vi "beads_DAQ_tmp.vi"() -> ()   [LabVIEW 2018]
panel:
  in  "Set Leak":bool
  out "apparent_leak_rate":dbl=8.332270636437045e-10
  in  "desired_leak_rate (torr*l/s)":dbl format="%.2e"
  out "P_baratron [torr]":dbl=6.441508062591926e-05 format="%#_3g"
  out "P_pirani [torr]":dbl=9.08455806667689e-05 format="%#_3g"
  out "P_1Tbaratro [torr]":dbl=8.203640319307528e-05 format="%#_3g"
  out "T_elec_rack [C]":dbl
  out "T_opt_table [C]":dbl
  in  "Read pressures?":bool=TRUE
  in  "Read temps?":bool
  in  "img_cluster":cluster{"Take Pic?":bool, "Only Images":bool}
  in  "Picomotor Stepping":T1={"Motor 1 Step Size"=-2, "zig zag iterations"=0, "Motor 2 Step Size"=0, "Step Picomotors?"=FALSE, "td (ms)"=0.0, "num"=0}
  in  "signal type":T2(ring)
  in  "Add small amp?":bool
  in  "Small amp freq (Hz)":dbl=10.0 format="%0.2p"
  in  "Small amp":dbl=1.0 format="%0.2p"
  in  "Flash lamp\n settings:":T3={"Flash lamp?"=FALSE, "Number of cyles\nbetween flashes"=2, "# Pulses"=2, "Stop flashing \nbelow thresh?"=TRUE, "Stop threshold"=25.0, "Pulse voltage?"=FALSE, "Pulse length (ms)"=0.001, "Pulse amp (V)"=0.001, "Disable AWG"=FALSE}
  in  "Stage settings:":T4={"Set stage?"=FALSE, "start X (um)"=40.0, "stop X (um) "=40.0, "# X Steps"=1, "start Y (um)"=40.0, "stop Y (um) "=40.0, "# Y steps"=1, "start Z (um)"=80.0, "stop Z (um)"=80.0, "# Z steps "=1, "Swp X?"=FALSE, "Amplitude X (um)"=40.0, "Frequency X (Hz)"=10.0, "Amplitude Y (um)"=40.0, "Frequency Y (Hz)"=3.7, "Amplitude Z (um)"=10.0, "Frequency Z (Hz)"=17.0, "Swp Y?"=FALSE, "Swp Z?"=FALSE}
  in  "Electrode settings:":T5={"DC volts (V):\n"=[0.0, 0.0, 0.0, 0.0, 0.0, 0.0, 0.0, 0.0], "Electrode to sweep:"=3, "start volt (V)"=4.0, "stop volt (V) "=4.0, "# V Steps"=1, "start freq (Hz)"=41.0, "stop freq (Hz) "=41.0, "# F steps"=1, "start DC (V)"=0.0, "stop DC (V)"=0.0, "# DC steps "=1, "Digitize electrode\ndrives?"=TRUE, "Sweep electrode?"=FALSE, "Add 0.5*V DC \noffset for amp?"=FALSE, "Use electrode \nconfig file?"=FALSE, "Path"=path "C:/GitHub/opt_lev/labview/DAQ_settings/electrode_sweep.txt", "Use arbitrary\nforce func?"=FALSE, "Voltage vs pos file"=path "C:/GitHub/opt_lev/labview/DAQ_settings/electrode_sweep.txt", "Use Arbitray\nelec drive"=FALSE, "Elec Drive File"=path "C:/GitHub/opt_lev_controls/labview/DAQ_settings/freq_comb_elec3_10V_1-600Hz_nocutsamp.txt", "Filter Elecs?"=FALSE, "Filter Cantilever?"=FALSE, "Control DDS"=TRUE, "x bias start (V)"=0.02, "x bias stop (V)"=-0.02, "y bias start (V)"=0.0, "y bias stop (V)"=0.0, "z bias start (V)"=0.0, "z bias stop (V)"=0.0}
  in  "DC supply settings:":T6
  out "Data":dbl[][](graph)
  out "Curr threshold":dbl=0.44040576014655786
  in  "Number of Samples":i32=50000
  in  "Sample Rate [Hz]":dbl=5000.0
  out "Actual Sample \nRate":dbl=5000.0 format="%0.2f"
  in  "Delay between files [s]":dbl=4.0 caption="Delay Time (s)"
  in  "Num files":i32=500
  in  "File base name":string="turbombar_powfb_xyzcool"
  in  "Directory path":path=path "D:/data/20210521/bead1/neutrality/w_height_fb_100V_41_Hz_bias_sweep_y_slow_dds_100kHz_spinning_xz"
  # "Logging Settings"
  # "Environment"
  # "Picomotor Stepping"
  # "Flash Lamp Settings"
  # "1: -35, 2: -30\n\n1: 32  2: 30"
  # "0"
  # "1"
  # "2"
  # "3"
  # "4"
  # "5"
  # "6"
  # "7"
  # "Acquired Data"
  # "Timing Settings"
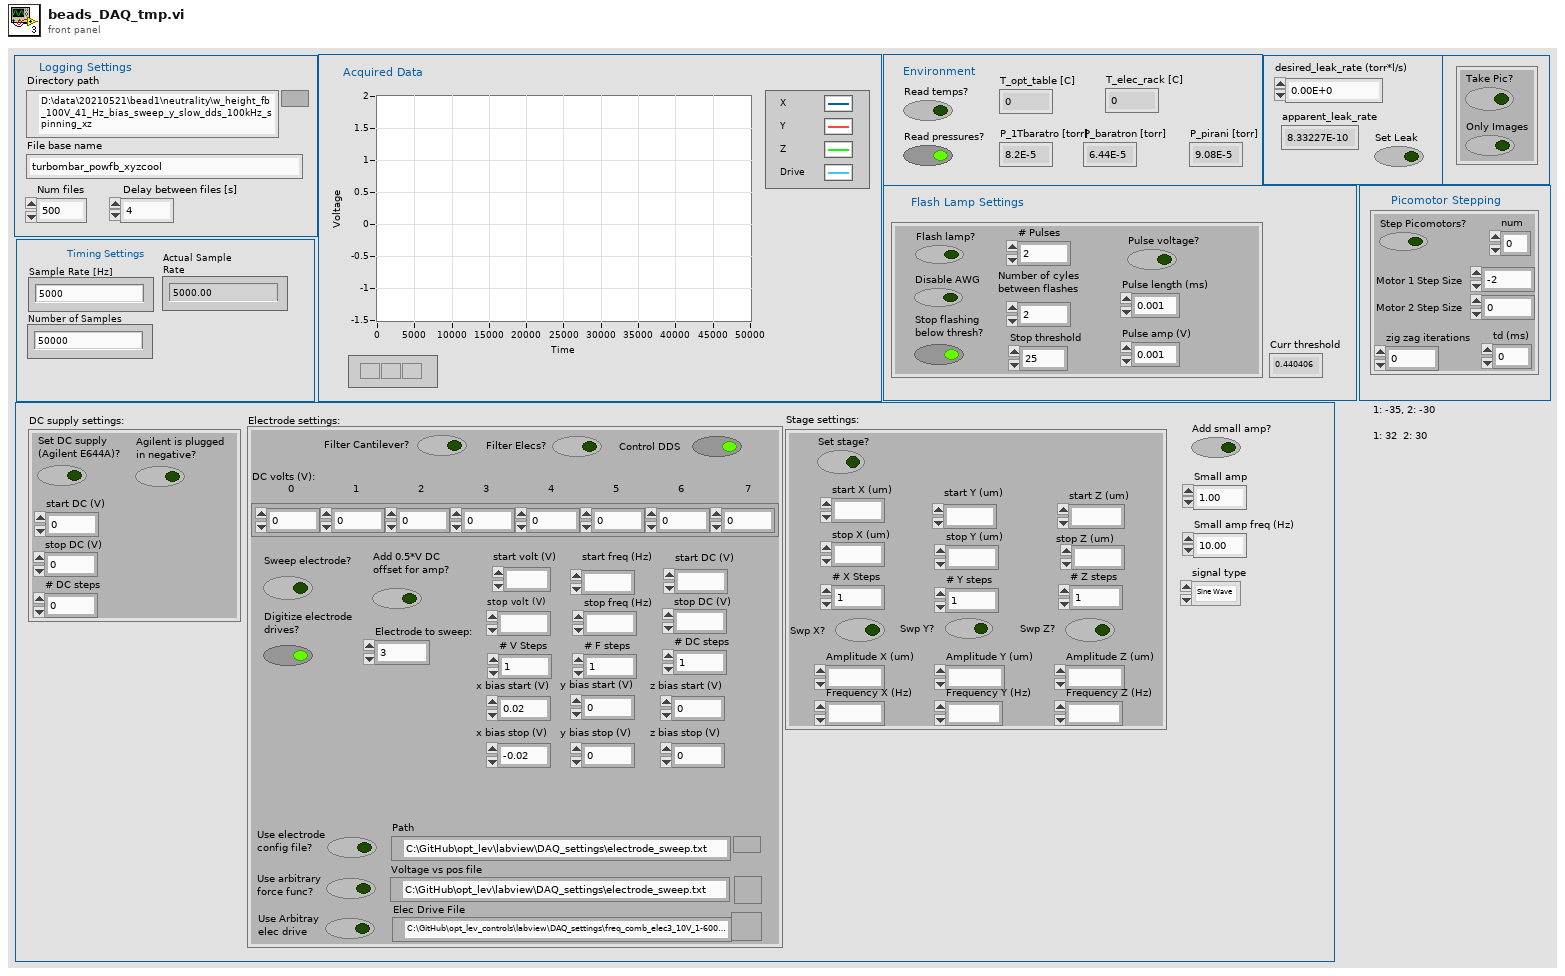
[diagram p1: front panel]
types:
  T1 = cluster{"Motor 1 Step Size":i32, "zig zag iterations":i32, "Motor 2 Step Size":i32, "Step Picomotors?":bool, "td (ms)":dbl, "num":i32}
  T2 = enum16{"Sine Wave", "Triangle Wave", "Square Wave", "Sawtooth Wave"}
  T3 = cluster{"Flash lamp?":bool, "Number of cyles\nbetween flashes":i32, "# Pulses":i32, "Stop flashing \nbelow thresh?":bool, "Stop threshold":dbl, "Pulse voltage?":bool, "Pulse length (ms)":dbl, "Pulse amp (V)":dbl, "Disable AWG":bool}
  T4 = cluster{"Set stage?":bool, "start X (um)":ext, "stop X (um) ":ext, "# X Steps":i32, "start Y (um)":ext, "stop Y (um) ":ext, "# Y steps":i32, "start Z (um)":ext, "stop Z (um)":ext, "# Z steps ":i32, "Swp X?":bool, "Amplitude X (um)":ext, "Frequency X (Hz)":ext, "Amplitude Y (um)":ext, "Frequency Y (Hz)":ext, "Amplitude Z (um)":ext, "Frequency Z (Hz)":ext, "Swp Y?":bool, "Swp Z?":bool}
  T5 = cluster{"DC volts (V):\n":dbl[], "Electrode to sweep:":i32, "start volt (V)":ext, "stop volt (V) ":ext, "# V Steps":i32, "start freq (Hz)":ext, "stop freq (Hz) ":ext, "# F steps":i32, "start DC (V)":ext, "stop DC (V)":ext, "# DC steps ":i32, "Digitize electrode\ndrives?":bool, "Sweep electrode?":bool, "Add 0.5*V DC \noffset for amp?":bool, "Use electrode \nconfig file?":bool, "Path":path, "Use arbitrary\nforce func?":bool, "Voltage vs pos file":path, "Use Arbitray\nelec drive":bool, "Elec Drive File":path, "Filter Elecs?":bool, "Filter Cantilever?":bool, "Control DDS":bool, "x bias start (V)":dbl, "x bias stop (V)":dbl, "y bias start (V)":dbl, "y bias stop (V)":dbl, "z bias start (V)":dbl, "z bias stop (V)":dbl}
  T6 = cluster{"start DC (V)":ext, "stop DC (V)":ext, "# DC steps ":i32, "Set DC supply\n(Agilent E644A)? ":bool, "Agilent is plugged \nin negative?":bool}
  T7 = cluster{"Number of Samples":i32, "Sample Rate [Hz]":dbl, "analog_input_channels":tag, "ref_clock_source":tag}
  T8 = cluster{"Tot DC Arr":dbl[], "Tot Electrode Arr":dbl[], "Tot Stage Arr":dbl[]}[]
  T9 = cluster{"analog_out_task":refnum<k21>, "analog_out_task_error":errorcluster}
  T10 = cluster{"CmdLib Out":refnum<k24>, "DeviceKey Out":string, "Device Address":i32, "error out":errorcluster}
  T11 = cluster{"Picomotor Instr":cluster{"CmdLib Out":refnum<k24>, "DeviceKey Out":string, "Device Address":i32, "error out":errorcluster}, "Picomotor Stepping":cluster{"Motor 1 Step Size":i32, "zig zag iterations":i32, "Motor 2 Step Size":i32, "Step Picomotors?":bool, "td (ms)":dbl, "num":i32}}
  T12 = cluster{"Output channel (for flashing)":tag, "Loop Iteration":i32, "path out":path, "Flash lamp\n settings:":cluster{"Flash lamp?":bool, "Number of cyles\nbetween flashes":i32, "# Pulses":i32, "Stop flashing \nbelow thresh?":bool, "Stop threshold":dbl, "Pulse voltage?":bool, "Pulse length (ms)":dbl, "Pulse amp (V)":dbl, "Disable AWG":bool}}
  T13 = enum16{"open", "replace", "create", "open or create", "replace or create", "replace or create with confirmation"}
  T14 = cluster{"CmdLib Out":refnum<k24>, "DeviceKey Out":string, "Device Address Out":i32, "error out":errorcluster, "Step Picomotors?":bool}
  T15 = cluster{"appended path":path, "base_path":path, "filename":string}
  T16 = cluster{"Agilent is \nplugged in \nnegative?":bool, "Set DC?":bool, "analog_out_task":refnum<k21>, "analog_out_task_error":errorcluster}
  T17 = cluster{"analog_input_task":refnum<k21>, "analog_input_task_error":errorcluster, "Actual Sample Rate (Hz)":dbl}
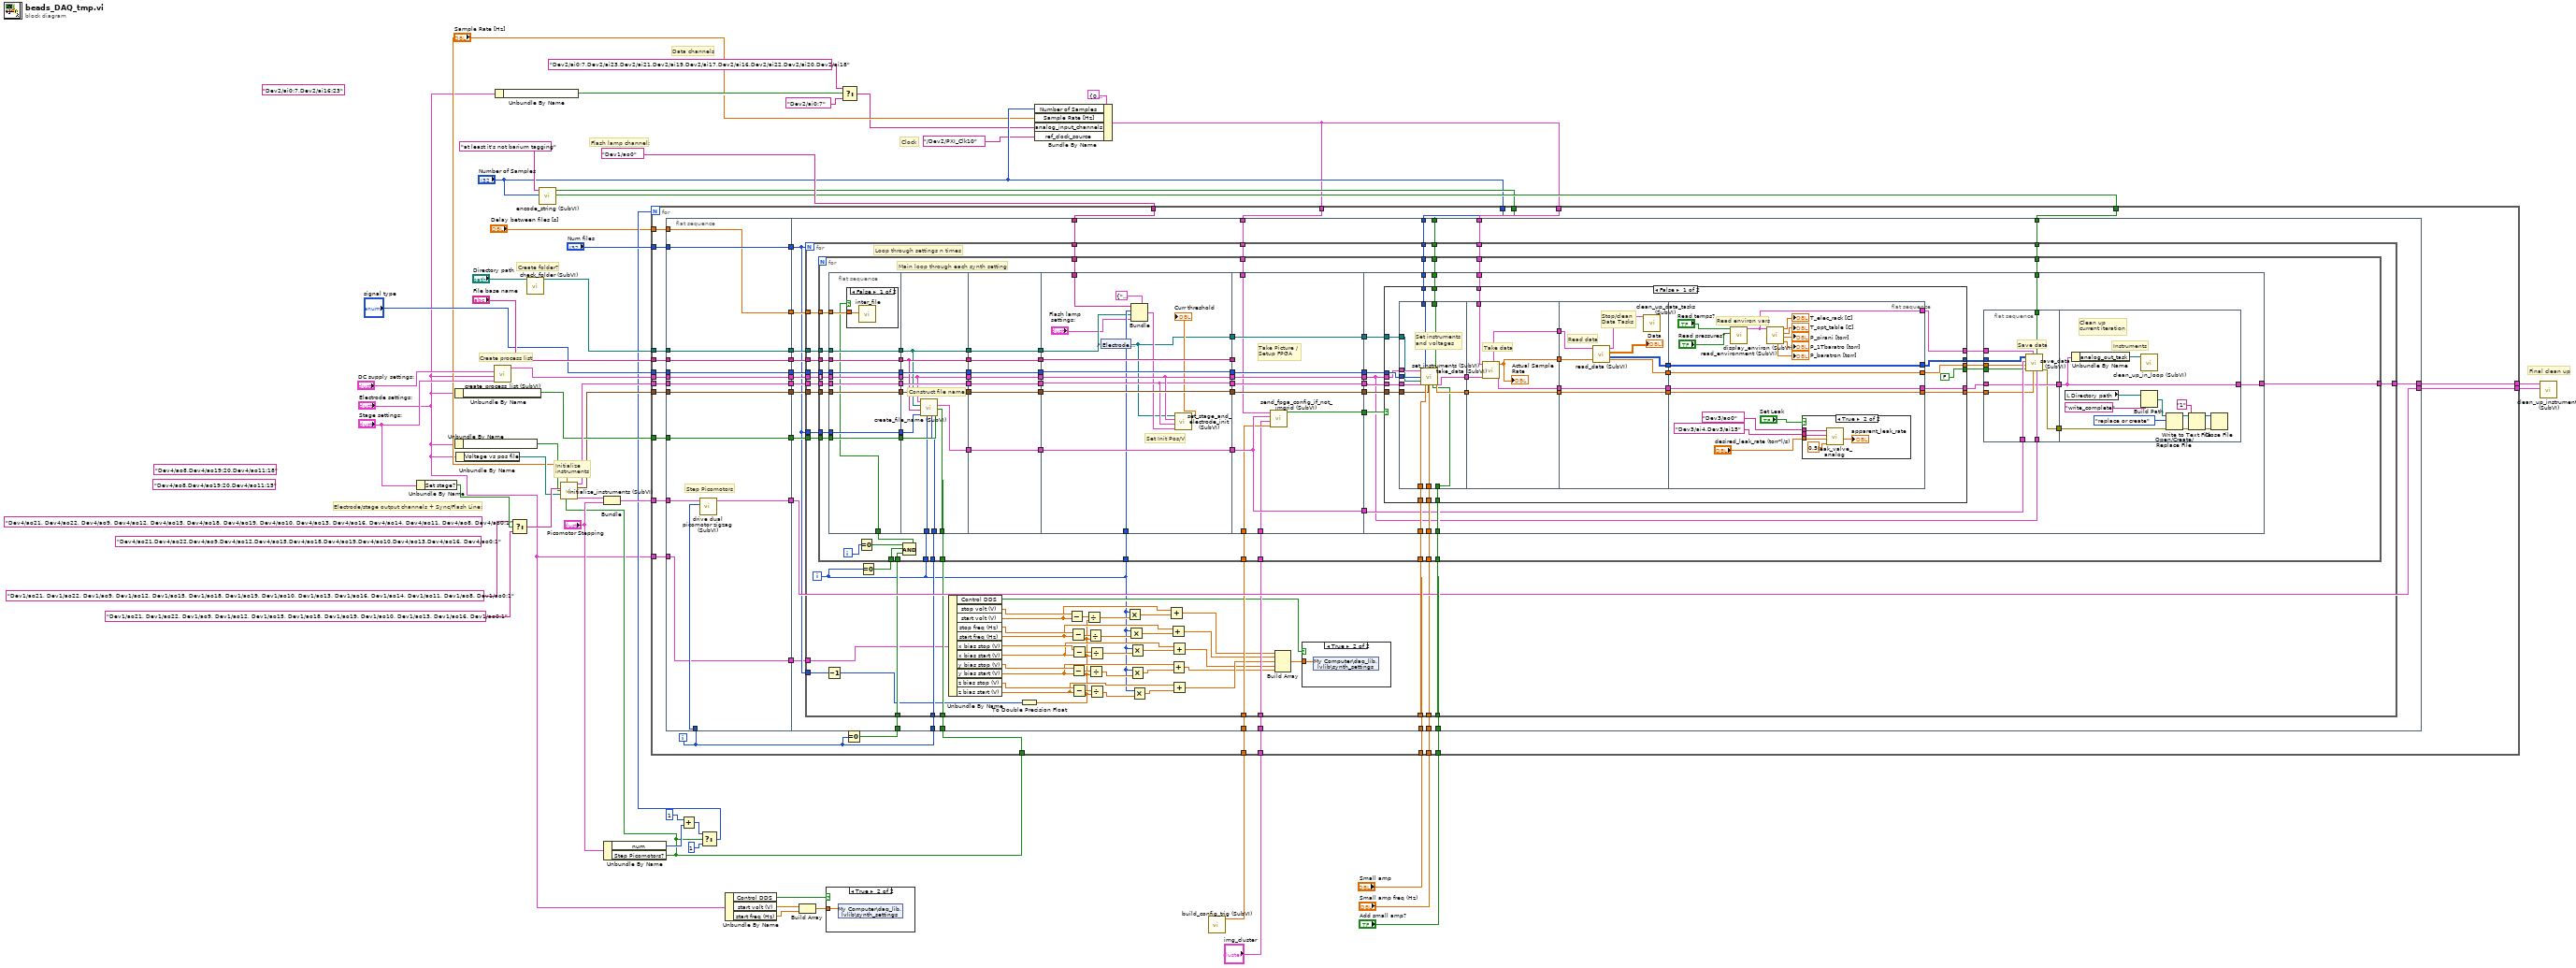
[diagram p0: block diagram]
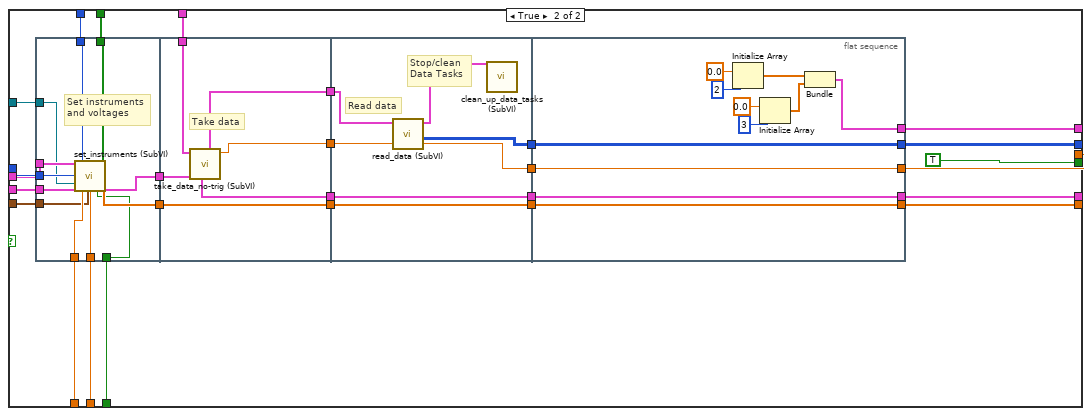
[diagram p6: hidden frame]
diagram:
  (unwired) tag "Dev4/ao21, Dev4/ao22, Dev4/ao9, Dev4/ao12, Dev4/ao15, Dev4/ao18, Dev4/ao19, Dev4/ao10, Dev4/ao13, Dev4/ao16, Dev4/ao14, Dev4/ao11, Dev4/ao8, Dev4/ao0:1" ("Output channel (for flashing)")
  (unwired) tag "Dev4/ao21,Dev4/ao22,Dev4/ao9,Dev4/ao12,Dev4/ao15,Dev4/ao18,Dev4/ao19,Dev4/ao10,Dev4/ao13,Dev4/ao16, Dev4/ao0:1" ("Output channel (for flashing)")
  (unwired) tag "Dev4/ao8,Dev4/ao19:20,Dev4/ao11:18" ("Output channel (for flashing)")
  (unwired) tag "Dev2/ai0:7,Dev2/ai16:23" ("Physical Channels (Position signals)")
  (unwired) tag "Dev4/ao8,Dev4/ao19:20,Dev4/ao11:15" ("Output channel (for flashing)")
  # "Final clean up"
  # "Clock"
  # "Data channels"
  # "Initialize\ninstruments"
  # "Electrode/stage output channels + Sync/Flash Line:"
  # "Flash lamp channel:"
  # "Create process list"
  # "Create folder?"
  n1 = Unbundle By Name("Stage settings:") -> ("Set stage?"=w42:bool)
  n2 = Unbundle By Name("Electrode settings:") -> ("Use electrode \nconfig file?"=w40:bool)
  n3 = Unbundle By Name("Electrode settings:") -> ("Use arbitrary\nforce func?"=w36:bool)
  n4 = Unbundle By Name("Electrode settings:") -> ("Voltage vs pos file"=w35:path)
  n5 = call "create_process_list (SubVI).vi"("DC supply settings:"="DC supply settings:", "Electrode settings: 2"="Electrode settings:", "Stage settings:"="Stage settings:") -> ("process_list"=w51:T8)  [unwired: 6 in]
  n6 = Unbundle By Name("Electrode settings:") -> ("Digitize electrode\ndrives?"=w44:bool)
  n7 = Select(t=tag "Dev1/ao21, Dev1/ao22, Dev1/ao9, Dev1/ao12, Dev1/ao15, Dev1/ao18, Dev1/ao19, Dev1/ao10, Dev1/ao13, Dev1/ao16, Dev1/ao14, Dev1/ao11, Dev1/ao8, Dev1/ao0:1" ("Output channel (for flashing)"), s=w42, f=tag "Dev1/ao21, Dev1/ao22, Dev1/ao9, Dev1/ao12, Dev1/ao15, Dev1/ao18, Dev1/ao19, Dev1/ao10, Dev1/ao13, Dev1/ao16, Dev1/ao0:1" ("Output channel (for flashing)")) -> (s? t:f=w41:tag)
  n8 = call "check_folder (SubVI).vi"("path in"="Directory path") -> ("path out"=w50:path)  [unwired: 10 in]
  n9 = call "encode_string (SubVI).vi"("nsamp"="Number of Samples", "encode_string"="at least it's not barium tagging") -> ("encoded_cropped"=w17:bool[], "encoded_out"=w15:bool[])  [unwired: 8 in]
  n10 = Unbundle By Name("Picomotor Stepping") -> ("num"=w23:i32, "Step Picomotors?"=w21:bool)
  n11 = call "initialize_instruments (SubVI).vi"("Sample rate"="Sample Rate [Hz]", "Electrode outupt channels"=w41, "make volt file"=w36, "volt file path"=w35, "Step Picomotors?"=w21) -> ("analog_out_config"=w49:T9, "Volt vs pos array"=w34:cluster{dbl, dbl}[], "Picomotor Instr"=w28:T10)  [unwired: 8 in]
  n12 = Bundle("Picomotor Instr"=w28, "Picomotor Stepping"="Picomotor Stepping") -> (w27:T11)  [unwired: 1 in]
  n13 = Add(x=1, y=w23) -> (x+y=w22:i32)
  n14 = Select(t=w22, s=w21, f=1) -> (s? t:f=w26:i32)
  n15 = Unbundle By Name("Electrode settings:") -> ("Control DDS"=w1:bool, "start volt (V)"=w11:ext, "start freq (Hz)"=w10:ext)
  n16 = Build Array(w11, w10) -> (w9:ext[])
  n17 = case shown="True" w1 {
    tunnel: w9 -> [_ w53]
    frame False {
    }
    frame True {
      n18 = shared-variable "My Computer\\daq_lib.lvlib\\synth_settings"(w53) -> ()  [unwired: 1 in, 1 out]
    }
  }
  n19 = Select(t=tag "Dev2/ai0:7,Dev2/ai23,Dev2/ai21,Dev2/ai19,Dev2/ai17,Dev2/ai16,Dev2/ai22,Dev2/ai20,Dev2/ai18" ("Physical Channels (Position signals)"), s=w44, f=tag "Dev2/ai0:7" ("Physical Channels (Position signals)")) -> (s? t:f=w5:tag)
  n20 = Bundle By Name(cluster=T7 {"Number of Samples"=0, "Sample Rate [Hz]"=0.0, "analog_input_channels"="", "ref_clock_source"=""} ("output cluster"), "Number of Samples"="Number of Samples", "Sample Rate [Hz]"="Sample Rate [Hz]", "analog_input_channels"=w5, "ref_clock_source"=tag "/Dev2/PXI_Clk10" ("Sample Clock Source")) -> (w3:T7)
  n21 = call "build_config_trig (SubVI).vi"() -> ("config_trig"=w14:dbl[])  [unwired: 11 in]
  n22 = for {
    N: w26 -> [_]
    tunnel: w51 -> [w91]
    tunnel: w50 -> [w90]
    tunnel: w49 -> [w89]
    tunnel: "Num files" -> [w88]
    tunnel: "File base name" -> [w87]
    tunnel: w3 -> [w86]
    tunnel: [w85] -> w46
    tunnel: "Number of Samples" -> [w84]
    tunnel: w40 -> [w83]
    tunnel: "Small amp" -> [w82]
    tunnel: "Small amp freq (Hz)" -> [w81]
    tunnel: "Add small amp?" -> [w80]
    tunnel: w34 -> [w79]
    tunnel: tag "Dev1/ao0" ("Output channel (for flashing)") -> [w78]
    tunnel: "signal type" -> [w77]
    tunnel: [w75] -> w30
    tunnel: w27 -> [w76]
    tunnel: w21 -> [w65]
    tunnel: "img_cluster" -> [w64]
    tunnel: w17 -> [w63]
    tunnel: "Delay between files [s]" -> [w61]
    tunnel: w15 -> [w60]
    tunnel: w3 -> [w59]
    tunnel: w14 -> [w58]
    tunnel: "Electrode settings:" -> [w55]
    i -> [w57]
    n23 = flat-sequence {
      tunnel: w76 -> [w96]
      tunnel: w77 -> [w97]
      tunnel: w79 -> [w98]
      tunnel: w83 -> [w99]
      tunnel: w87 -> [w100]
      tunnel: w88 -> [w101]
      tunnel: w89 -> [w102]
      tunnel: w90 -> [w103]
      tunnel: w91 -> [w104]
      tunnel: [w104] -> w74
      tunnel: [w103] -> w73
      tunnel: [w102] -> w72
      tunnel: [w101] -> w71
      tunnel: [w100] -> w70
      tunnel: [w99] -> w69
      tunnel: [w98] -> w68
      tunnel: [w97] -> w67
      tunnel: [w95] -> w66
      tunnel: w57 -> [w94]
      tunnel: [w93] -> w62
      tunnel: w61 -> [w93]
      tunnel: w55 -> [w92]
      tunnel: [w92] -> w54
      tunnel: w86 -> [w126]
      tunnel: [w125] -> w85
      tunnel: w84 -> [w124]
      tunnel: w82 -> [w122]
      tunnel: w81 -> [w121]
      tunnel: w80 -> [w120]
      tunnel: w78 -> [w118]
      tunnel: [w116] -> w75
      tunnel: w74 -> [w130]
      tunnel: w73 -> [w129]
      tunnel: w72 -> [w128]
      tunnel: w71 -> [w106]
      tunnel: w70 -> [w127]
      tunnel: w69 -> [w123]
      tunnel: w68 -> [w119]
      tunnel: w67 -> [w117]
      tunnel: w66 -> [w116]
      tunnel: w57 -> [w115]
      tunnel: w65 -> [w114]
      tunnel: w64 -> [w113]
      tunnel: w63 -> [w112]
      tunnel: w62 -> [w111]
      tunnel: w60 -> [w110]
      tunnel: w59 -> [w109]
      tunnel: w58 -> [w108]
      tunnel: w56 -> [w107]
      tunnel: w54 -> [w105]
      frame #0 {
        # "Step Picomotors"
        n24 = call "drive dual picomotor zigzag (SubVI).vi"("Picomotor Index"=w94, "Picomotor Cluster"=w96) -> ("Picomotor Instr Out"=w95:T14)  [unwired: 9 in]
      }
      frame #1 {
        n25 = for {
          N: w106 -> [_]
          tunnel: w130 -> [w192]
          tunnel: w118 -> [w172]
          tunnel: w129 -> [w191]
          tunnel: w128 -> [w190]
          tunnel: w106 -> [w189]
          tunnel: w127 -> [w188]
          tunnel: w126 -> [w187]
          tunnel: [w186] -> w125
          tunnel: w124 -> [w185]
          tunnel: w123 -> [w184]
          tunnel: w122 -> [w183]
          tunnel: w121 -> [w182]
          tunnel: w120 -> [w181]
          tunnel: w119 -> [w180]
          tunnel: w117 -> [w179]
          tunnel: w115 -> [w178]
          tunnel: w114 -> [w177]
          tunnel: w113 -> [w176]
          tunnel: w112 -> [w175]
          tunnel: w111 -> [w174]
          tunnel: w110 -> [w173]
          tunnel: w109 -> [w171]
          tunnel: w108 -> [w170]
          tunnel: w107 -> [w168]
          tunnel: w106 -> [w166]
          tunnel: w105 -> [w161]
          i -> [w134]
          # "Loop through settings n times"
          n26 = Decrement(x=w166) -> (x-1=w160:i32)
          n27 = Equal To 0?(x=w134) -> (x = 0?=w169:bool)
          n28 = for {
            tunnel: w192 -> [w246] mode=indexing
            tunnel: w191 -> [w259]
            tunnel: w190 -> [w258]
            tunnel: w189 -> [w257]
            tunnel: w188 -> [w256]
            tunnel: w187 -> [w255]
            tunnel: [w254] -> w186
            tunnel: w185 -> [w253]
            tunnel: w184 -> [w252]
            tunnel: w183 -> [w251]
            tunnel: w182 -> [w250]
            tunnel: w181 -> [w249]
            tunnel: w180 -> [w248]
            tunnel: w179 -> [w247]
            tunnel: w178 -> [w230]
            tunnel: w177 -> [w229]
            tunnel: w134 -> [w231]
            tunnel: w176 -> [w209]
            tunnel: w175 -> [w232]
            tunnel: w174 -> [w220]
            tunnel: w173 -> [w219]
            tunnel: w172 -> [w218]
            tunnel: w134 -> [w217]
            tunnel: w171 -> [w216]
            tunnel: w170 -> [w194]
            tunnel: w169 -> [w213]
            tunnel: w168 -> [w212]
            i -> [w215]
            # "Main loop through each synth setting"
            n29 = flat-sequence {
              tunnel: w247 -> [w262]
              tunnel: w248 -> [w263]
              tunnel: w252 -> [w264]
              tunnel: w256 -> [w265]
              tunnel: w257 -> [w266]
              tunnel: w258 -> [w267]
              tunnel: w259 -> [w268]
              tunnel: w246 -> [w269]
              tunnel: [w269] -> w228
              tunnel: [w268] -> w227
              tunnel: [w267] -> w226
              tunnel: [w266] -> w225
              tunnel: [w265] -> w224
              tunnel: [w264] -> w223
              tunnel: [w263] -> w222
              tunnel: [w262] -> w221
              tunnel: w220 -> [w261]
              tunnel: w211 -> [w260]
              tunnel: [w277] -> w208
              tunnel: [w278] -> w206
              tunnel: [w282] -> w204
              tunnel: [w279] -> w202
              tunnel: [w281] -> w200
              tunnel: [w280] -> w198
              tunnel: [w271] -> w196
              tunnel: w231 -> [w274]
              tunnel: w230 -> [w273]
              tunnel: w229 -> [w272]
              tunnel: w228 -> [w277]
              tunnel: w227 -> [w278]
              tunnel: w226 -> [w282]
              tunnel: w225 -> [w276]
              tunnel: w224 -> [w279]
              tunnel: w223 -> [w275]
              tunnel: w222 -> [w281]
              tunnel: w221 -> [w280]
              tunnel: w208 -> [w283]
              tunnel: [w283] -> w207
              tunnel: w206 -> [w289]
              tunnel: [w289] -> w205
              tunnel: w204 -> [w288]
              tunnel: [w288] -> w203
              tunnel: w202 -> [w287]
              tunnel: [w287] -> w201
              tunnel: w200 -> [w286]
              tunnel: [w286] -> w199
              tunnel: w198 -> [w285]
              tunnel: [w285] -> w197
              tunnel: w196 -> [w284]
              tunnel: [w284] -> w195
              tunnel: [w301] -> w245
              tunnel: [w300] -> w243
              tunnel: [w303] -> w241
              tunnel: [w302] -> w239
              tunnel: [w290] -> w237
              tunnel: [w299] -> w235
              tunnel: [w298] -> w233
              tunnel: w207 -> [w301]
              tunnel: w205 -> [w295]
              tunnel: w203 -> [w300]
              tunnel: w201 -> [w299]
              tunnel: w199 -> [w303]
              tunnel: w197 -> [w302]
              tunnel: w195 -> [w298]
              tunnel: w218 -> [w297]
              tunnel: w217 -> [w296]
              tunnel: w245 -> [w313]
              tunnel: [w313] -> w244
              tunnel: w243 -> [w312]
              tunnel: [w312] -> w242
              tunnel: w241 -> [w311]
              tunnel: [w311] -> w240
              tunnel: w239 -> [w310]
              tunnel: [w310] -> w238
              tunnel: w237 -> [w309]
              tunnel: [w309] -> w236
              tunnel: w235 -> [_]
              tunnel: [w307] -> w234
              tunnel: w233 -> [w307]
              tunnel: w216 -> [w308]
              tunnel: w194 -> [w306]
              tunnel: [w304] -> w210
              tunnel: w209 -> [w305]
              tunnel: w255 -> [w336]
              tunnel: w219 -> [w327]
              tunnel: w234 -> [w325]
              tunnel: w236 -> [w328]
              tunnel: w238 -> [w329]
              tunnel: w240 -> [w330]
              tunnel: w242 -> [w335]
              tunnel: w244 -> [w324]
              tunnel: w249 -> [w331]
              tunnel: w250 -> [w332]
              tunnel: w251 -> [w333]
              tunnel: w253 -> [w334]
              tunnel: w232 -> [w319]
              tunnel: w210 -> [w326]
              tunnel: [w317] -> w254
              frame #0 {
                n30 = case shown="False" w260 {
                  tunnel: w261 -> [w270 _]
                  frame False {
                    n31 = call "inter_file"("Delay Time (s)"=w270) -> ()  [unwired: 10 in, 1 out]
                  }
                  frame True {
                  }
                }
              }
              frame #1 {
                # "Construct file name"
                n32 = call "create_file_name (SubVI).vi"("Use electrode config?"=w275, "Step Picomotors?"=w272, "picomotor index"=w273, "file_idx"=w274, "num files"=w276, "base name"=w279, "Path"=w278, "process_list"=w277) -> ("filename_cluster"=w271:T15)  [unwired: 3 in]
              }
              frame #2 {
              }
              frame #3 {
                # "Set Init Pos/V"
                n33 = control-ref of="Electrode settings:"() -> (w290:refnum<vi>)
                n34 = Bundle(cluster=T12 {"Output channel (for flashing)"="", "Loop Iteration"=0, "path out"=path "", "Flash lamp\n settings:"={"Flash lamp?"=FALSE, "Number of cyles\nbetween flashes"=0, "# Pulses"=0, "Stop flashing \nbelow thresh?"=FALSE, "Stop threshold"=0.0, "Pulse voltage?"=FALSE, "Pulse length (ms)"=0.0, "Pulse amp (V)"=0.0, "Disable AWG"=FALSE}} ("output cluster"), "Output channel (for flashing)"=w297, "Loop Iteration"=w296, "path out"=w295, "Flash lamp\n settings:"="Flash lamp\n settings:") -> (w291:T12)
                n35 = call "set_stage_and_electrode_init (SubVI).vi"("output cluster"=w291, "instrument config"=w300, "Process list"=w301, "Cluster in"=w290) -> ("Curr threshold"=→"Curr threshold":dbl)  [unwired: 7 in]
              }
              frame #4 {
                # "Take Picture / \nSetup FPGA"
                n36 = call "send_fpga_config_if_not_imgrid (SubVI).vi"("config_trig"=w306, "img_cluster"=w305, "file_path_cluster"=w307, "channel_settings"=w308) -> ("Only Images"=w304:bool)  [unwired: 7 in]
              }
              frame #5 {
                n37 = case shown="False" w326 {
                  tunnel: [w359 w437] -> w318
                  tunnel: w324 -> [w365 w438]
                  tunnel: w336 -> [w374 w447]
                  tunnel: w335 -> [w385 w458]
                  tunnel: w334 -> [w384 w457]
                  tunnel: w333 -> [w383 w456]
                  tunnel: w332 -> [w382 w455]
                  tunnel: w331 -> [w381 w454]
                  tunnel: w330 -> [w380 w453]
                  tunnel: w329 -> [w379 w452]
                  tunnel: w328 -> [w378 w451]
                  tunnel: w327 -> [w377 w450]
                  tunnel: [w364 w436] -> w323
                  tunnel: [w363 w432] -> w322
                  tunnel: [w362 w435] -> w321
                  tunnel: [w361 w434] -> w320
                  tunnel: [FALSE TRUE] -> w315
                  frame False {
                    n38 = flat-sequence {
                      tunnel: w365 -> [w397]
                      tunnel: w385 -> [w395]
                      tunnel: w384 -> [w394]
                      tunnel: w383 -> [w393]
                      tunnel: w382 -> [w392]
                      tunnel: w381 -> [w391]
                      tunnel: w380 -> [w390]
                      tunnel: w379 -> [w389]
                      tunnel: w378 -> [w388]
                      tunnel: w377 -> [w387]
                      tunnel: [w396] -> w376
                      tunnel: [w386] -> w375
                      tunnel: w376 -> [w403]
                      tunnel: w375 -> [w401]
                      tunnel: w374 -> [w400]
                      tunnel: [w403] -> w373
                      tunnel: [w402] -> w372
                      tunnel: [w398] -> w371
                      tunnel: [w399] -> w370
                      tunnel: w373 -> [w410]
                      tunnel: w372 -> [w404]
                      tunnel: w371 -> [w409]
                      tunnel: w370 -> [w408]
                      tunnel: [w410] -> w369
                      tunnel: [w409] -> w368
                      tunnel: [w408] -> w367
                      tunnel: [w405] -> w366
                      tunnel: w369 -> [w426]
                      tunnel: w368 -> [w425]
                      tunnel: w367 -> [w424]
                      tunnel: w366 -> [w423]
                      tunnel: [w426] -> w364
                      tunnel: [w425] -> w359
                      tunnel: [w424] -> w361
                      tunnel: [w423] -> w362
                      tunnel: [w415] -> w363
                      frame #0 {
                        # "Set instruments\nand voltages"
                        n39 = call "set_instruments (SubVI).vi"("process_list"=w397, "signal type"=w389, "electrodes reference"=w388, "instrument config"=w395, "Num samples"=w394, "small amp"=w393, "Volt vs pos array"=w390, "small amp freq"=w392, "Add small amp?"=w391, "encode_bits"=w387) -> ("DC volts arr"=w396:dbl[], "instrument out"=w386:T16)  [unwired: 8 in]
                      }
                      frame #1 {
                        # "Take data"
                        n40 = call "take_data (SubVI).vi"("instrument in"=w401, "channel_settings"=w400) -> ("instrument out"=w398:T16, "Actual Sample Rate"=w399:dbl, "data_cluster"=w402:T17)  [unwired: 7 in]
                        "Actual Sample \nRate" <- w399
                      }
                      frame #2 {
                        # "Read data"
                        # "Stop/clean \nData Tasks"
                        n41 = call "read_data (SubVI).vi"("data_cluster_in"=w404) -> ("Rescaled data"=w405:i16[][], "Output data"=→"Data":dbl[][], "data_cluster_out"=w406:T17)  [unwired: 7 in, 1 out]
                        n42 = call "clean_up_data_tasks (SubVI).vi"("data_cluster"=w406) -> ()  [unwired: 11 in]
                      }
                      frame #3 {
                        # "Read environ vars"
                        n43 = call "read_environment (SubVI).vi"("Read pressures?"="Read pressures?", "Read temps?"="Read temps?") -> ("environ cluster"=w415:cluster{dbl[], dbl[]})  [unwired: 9 in]
                        n44 = call "display_environ (SubVI).vi"("environ cluster"=w415) -> ("P_pirani"=→"P_1Tbaratro [torr]":dbl, "P_cc"=→"P_pirani [torr]":dbl, "T_opt_table"=→"T_opt_table [C]":dbl, "T_elec_rack"=→"T_elec_rack [C]":dbl, "P_baratron"=→"P_baratron [torr]":dbl)  [unwired: 6 in]
                        n45 = case shown="True" "Set Leak" {
                          tunnel: "desired_leak_rate (torr*l/s)" -> [_ w431]
                          tunnel: tag "Dev3/ao0" ("leak_control_channel") -> [_ w430]
                          tunnel: tag "Dev3/ai4,Dev3/ai15" ("valve_pos_channel") -> [_ w429]
                          frame False {
                          }
                          frame True {
                            n46 = call "leak_valve_analog.vi"("read/write delay"=0.5, "desired_leak_rate (torr*l/s)"=w431, "valve_pos_channel"=w429, "leak_control_channel"=w430) -> ("apparent_leak_rate"=→"apparent_leak_rate":dbl)  [unwired: 4 in, 2 out]
                          }
                        }
                      }
                    }
                  }
                  frame True {
                    n47 = flat-sequence {
                      tunnel: w438 -> [w470]
                      tunnel: w458 -> [w467]
                      tunnel: w457 -> [w466]
                      tunnel: w456 -> [w465]
                      tunnel: w455 -> [w464]
                      tunnel: w454 -> [w463]
                      tunnel: w453 -> [w462]
                      tunnel: w452 -> [w461]
                      tunnel: w451 -> [w460]
                      tunnel: w450 -> [w459]
                      tunnel: [w469] -> w449
                      tunnel: [w468] -> w448
                      tunnel: w449 -> [w476]
                      tunnel: w448 -> [w474]
                      tunnel: w447 -> [w473]
                      tunnel: [w476] -> w446
                      tunnel: [w475] -> w445
                      tunnel: [w472] -> w444
                      tunnel: [w471] -> w443
                      tunnel: w446 -> [w482]
                      tunnel: w445 -> [w479]
                      tunnel: w444 -> [w481]
                      tunnel: w443 -> [w480]
                      tunnel: [w482] -> w442
                      tunnel: [w481] -> w441
                      tunnel: [w480] -> w440
                      tunnel: [w477] -> w439
                      tunnel: w442 -> [w493]
                      tunnel: w441 -> [w492]
                      tunnel: w440 -> [w491]
                      tunnel: w439 -> [w490]
                      tunnel: [w493] -> w436
                      tunnel: [w492] -> w437
                      tunnel: [w491] -> w434
                      tunnel: [w490] -> w435
                      tunnel: [w485] -> w432
                      frame #0 {
                        # "Set instruments\nand voltages"
                        n48 = call "set_instruments (SubVI).vi"("process_list"=w470, "signal type"=w461, "electrodes reference"=w460, "instrument config"=w467, "Num samples"=w466, "small amp"=w465, "Volt vs pos array"=w462, "small amp freq"=w464, "Add small amp?"=w463, "encode_bits"=w459) -> ("DC volts arr"=w469:dbl[], "instrument out"=w468:T16)  [unwired: 8 in]
                      }
                      frame #1 {
                        # "Take data"
                        n49 = call "take_data_no-trig (SubVI).vi"("instrument in"=w474, "channel_settings"=w473) -> ("Actual Sample Rate"=w471:dbl, "data_cluster"=w475:T17, "instrument out"=w472:T16)  [unwired: 7 in]
                      }
                      frame #2 {
                        # "Read data"
                        # "Stop/clean \nData Tasks"
                        n50 = call "read_data (SubVI).vi"("data_cluster_in"=w479) -> ("Rescaled data"=w477:i16[][], "data_cluster_out"=w478:T17)  [unwired: 7 in, 2 out]
                        n51 = call "clean_up_data_tasks (SubVI).vi"("data_cluster"=w478) -> ()  [unwired: 11 in]
                      }
                      frame #3 {
                        n52 = Initialize Array(0.0 ("element"), 2 ("dimension size")) -> (w484:dbl[])
                        n53 = Initialize Array(0.0 ("element"), 3 ("dimension size")) -> (w483:dbl[])
                        n54 = Bundle(w484, w483) -> (w485:cluster{dbl[], dbl[]})  [unwired: 1 in]
                      }
                    }
                  }
                }
                n55 = flat-sequence {
                  tunnel: w325 -> [w346]
                  tunnel: w324 -> [w345]
                  tunnel: w323 -> [w344]
                  tunnel: w322 -> [w343]
                  tunnel: w321 -> [w342]
                  tunnel: w320 -> [w341]
                  tunnel: w319 -> [w340]
                  tunnel: w318 -> [w339]
                  tunnel: [w339] -> w316
                  tunnel: w315 -> [w338]
                  tunnel: [w337] -> w314
                  tunnel: [w357] -> w317
                  tunnel: w316 -> [w357]
                  tunnel: w314 -> [w356]
                  frame #0 {
                    # "Save data"
                    n56 = call "save_data (SubVI).vi"("Process list"=w345, "encoded_bits"=w340, "DC volts arr"=w344, "environ cluster"=w343, "imgrid"=w338, "Fsamp"=w341, "file_path_cluster"=w346, "data"=w342) -> ("error out"=w337:errorcluster)  [unwired: 3 in]
                  }
                  frame #1 {
                    # "Clean up\ncurrent iteration"
                    # "Instruments"
                    n57 = local read "Directory path"() -> (w355:path)
                    n58 = Unbundle By Name(w357) -> ("analog_out_task"=w358:refnum<k21>)
                    n59 = Build Path(base path=w355, name or relative path="write_complete") -> (appended path=w353:path)
                    n60 = call "clean_up_in_loop (SubVI).vi"("Refnum in"=w358) -> ()  [unwired: 10 in, 1 out]
                    n61 = Open/Create/Replace File(file path (use dialog)=w353, error in=w356, operation (0:open)=T13."replace or create") -> (refnum out=w351:refnum<file>, error out=w352:errorcluster)  [unwired: 3 in, 1 out]
                    n62 = Write to Text File(file (use dialog)=w351, text="1", error in=w352) -> (refnum out=w347:refnum<file>, error out=w348:errorcluster)  [unwired: 1 in, 1 out]
                    n63 = Close File(refnum=w347, error in=w348) -> ()  [unwired: 2 out]
                  }
                }
              }
            }
            n64 = Equal To 0?(x=w215) -> (x = 0?=w214:bool)
            n65 = Compound Arithmetic op=AND(w214, w213, w212) -> (w211:bool)
          }
          n66 = Unbundle By Name(w161) -> ("Control DDS"=w135:bool, "stop volt (V)"=w139:ext, "start volt (V)"=w138:ext, "stop freq (Hz)"=w145:ext, "start freq (Hz)"=w144:ext, "x bias stop (V)"=w165:dbl, "x bias start (V)"=w150:dbl, "y bias stop (V)"=w153:dbl, "y bias start (V)"=w151:dbl, "z bias stop (V)"=w162:dbl, "z bias start (V)"=w154:dbl)
          n67 = To Double Precision Float(number=w160) -> (double precision float=w136:dbl)
          n68 = Subtract(x=w139, y=w138) -> (x-y=w141:ext)
          n69 = Subtract(x=w145, y=w144) -> (x-y=w147:ext)
          n70 = Subtract(x=w153, y=w151) -> (x-y=w164:dbl)
          n71 = Subtract(x=w165, y=w150) -> (x-y=w155:dbl)
          n72 = Subtract(x=w162, y=w154) -> (x-y=w163:dbl)
          n73 = Divide(x=w141, y=w136) -> (x/y=w142:ext)
          n74 = Divide(x=w147, y=w136) -> (x/y=w148:ext)
          n75 = Divide(x=w164, y=w136) -> (x/y=w158:dbl)
          n76 = Divide(x=w155, y=w136) -> (x/y=w156:dbl)
          n77 = Divide(x=w163, y=w136) -> (x/y=w159:dbl)
          n78 = Multiply(x=w134, y=w142) -> (x*y=w140:ext)
          n79 = Multiply(x=w134, y=w148) -> (x*y=w146:ext)
          n80 = Multiply(x=w134, y=w156) -> (x*y=w152:dbl)
          n81 = Multiply(x=w134, y=w158) -> (x*y=w149:dbl)
          n82 = Multiply(x=w134, y=w159) -> (x*y=w157:dbl)
          n83 = Add(x=w138, y=w140) -> (x+y=w137:ext)
          n84 = Add(x=w144, y=w146) -> (x+y=w143:ext)
          n85 = Add(x=w151, y=w149) -> (x+y=w131:dbl)
          n86 = Add(x=w150, y=w152) -> (x+y=w132:dbl)
          n87 = Add(x=w154, y=w157) -> (x+y=w133:dbl)
          n88 = Build Array(w137, w143, w133, w132, w131) -> (w167:ext[])
          n89 = case shown="True" w135 {
            tunnel: w167 -> [_ w193]
            frame False {
            }
            frame True {
              n90 = shared-variable "My Computer\\daq_lib.lvlib\\synth_settings"(w193) -> ()  [unwired: 1 in, 1 out]
            }
          }
        }
      }
    }
    n91 = Equal To 0?(x=w57) -> (x = 0?=w56:bool)
  }
  n92 = call "clean_up_instruments (SubVI).vi"("Picomotor Instr Out"=w30, "instrument in"=w46) -> ()  [unwired: 10 in]
